vi "General Error Handler CORE.vi"(0 "[error code] (0)":i32 format="%0.0f", 1 "[user-defined codes]":i32[](array[numeric]), 2 "[user-defined descriptions]":string[](array[string]), 5 "[error source] (\" \")":string, 7 "String to Format (not a refnum)":refnum<vi>, 9 "type of dialog (OK msg:1)":T2=enum."OK message", 11 "error in (no error)":errorcluster, 12 "[exception action] (none:0)":i32(ring) items=["no exception", "cancel error on match", "set error on match"], 13 "[exception code]":i32 format="%0.0f", 14 "[exception source]":string) -> (3 "stop event propagated":bool, 4 "error?":bool, 6 "code out":i32 format="%0.0f", 8 "source out":string, 10 "message":string=" INSTRUCTIONS:\r\rNormal Use:  When using subVIs that incorporate the error in/error out (or error I/O) structure, place this handler where you want to inform the user of an error, typically at the end of the I/O data path, as the last action of the program.  If the error in error? is ERROR, the handler creates a message describing the error and its source.  If the type of dialog = 1 (default), the message is displayed to the user, who can only acknowledge it.  If the type = 2, the user can acknowledge the message or abort execution; aborting a program with active I/O is not recommended.  If the type = 0, no message is displayed; this is used to process the error programmatically, and the error out cluster elements are wired to individual terminals for that reason.  \r\rOther Use:\n\r\nlocal testing.  To test the error code of a subVI or function that does not have the error I/O structure, you can wire its error code and a source string to the local error code and error source inputs.  If error in error? indicates no error and error code is not equal to 0, the local code and source are substituted for the error in values, and error? is set TRUE (ERROR).", 15 "error out":errorcluster)   [LabVIEW 2011]
doc: "Indicates whether an error occurred. If an error occurred, this VI returns a description of the error and optionally displays a dialog box."
uses:
  DialogTypeEnum.ctl
  whitespace.ctl
panel:
  in  "prompts":T1={"Error %d occurred at %s"="Error %d occurred at %s", "Warning %d occurred at %s"="Warning %d occurred at %s", "Possible reasons: %s"="<b>Possible reason(s):</b>\\n%s", "Error not listed"="This error code is undefined. Undefined errors might occur for a number of reasons. For example, no one has provided a description for the code, or you might have wired a number that is not an error code to the error code input. \n\nAdditionally, undefined error codes might occur because the error relates to a third-party object, such as the operating system or ActiveX. For these third-party errors, you might be able to obtain a description of the error by searching the Web for the error code (%s) or for its hexadecimal representation (0x%s).", "GetCommError x%lx"="Windows GetCommError:  The hex value of this code is <B>x%04lx</B>.\n\nInterpret it bit-wise as follows:\n<B>x4000</B>: serial port VI error\n<B>x0001</B>: receiving queue overflowed or character was received after end-of-file character\n<B>x0002</B>: character was lost by overwrite\n<B>x0004</B>: parity error\n<B>x0008</B>: framing error\n<B>x0010</B>: break condition\n<B>x0020</B>: CTS timeout\n<B>x0040</B>: DSR timeout\n<B>x0080</B>: RLSD timeout\n<B>x0100</B>: transmission queue was full when new character arrived\n<B>x0200</B>: parallel device timeout\n<B>x0400</B>: parallel device I/O error\n<B>x0800</B>: parallel device not selected\n<B>x1000</B>: parallel device out of paper\n<B>x8000</B>: requested mode is  not supported or the idComDev parameter is invalid.", "Continue"="Continue", "Stop"="Stop", "an unidentified location"="an unidentified location", "No Error"="No Error", "Help"="Why not found?"}
  # "reinitialize to default to display instructions"
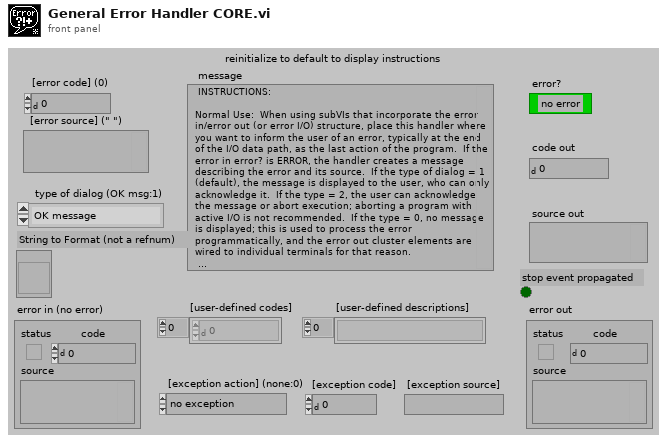
[diagram p1: front panel]
types:
  T1 = cluster{"Error %d occurred at %s":string, "Warning %d occurred at %s":string, "Possible reasons: %s":string, "Error not listed":string, "GetCommError x%lx":string, "Continue":string, "Stop":string, "an unidentified location":string, "No Error":string, "Help":string}
  T2 = typedef "DialogTypeEnum.ctl" = enum16{"no dialog", "OK message", "continue or stop message", "auto error handling dialog", "OK message + warnings", "continue/stop + warnings"}
  T3 = typedef "TagReturnType.ctl" = enum16{"No Tag", "<err>", "<append>"}
  T4 = typedef "whitespace.ctl" = u16
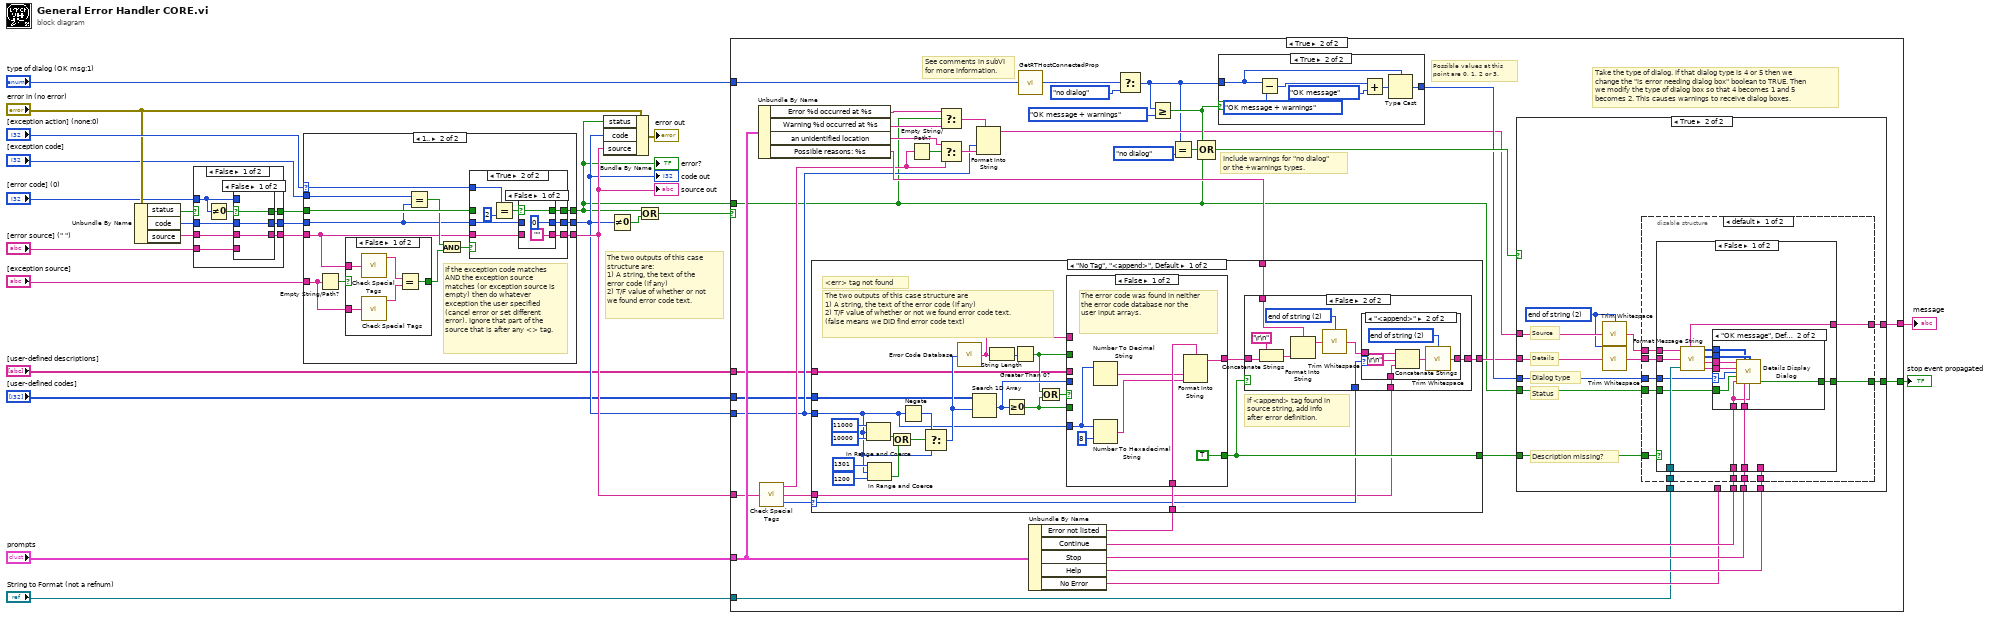
[diagram p0: block diagram]
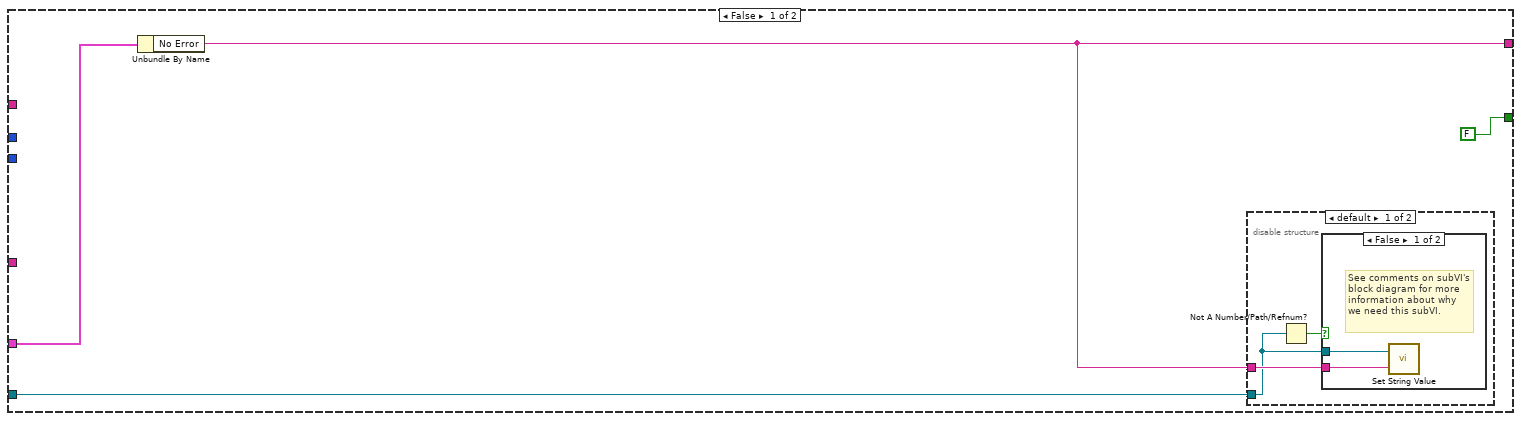
[diagram p8: hidden frame]
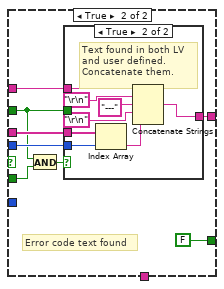
[diagram p14: hidden frame]
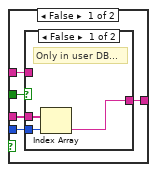
[diagram p15: hidden frame]
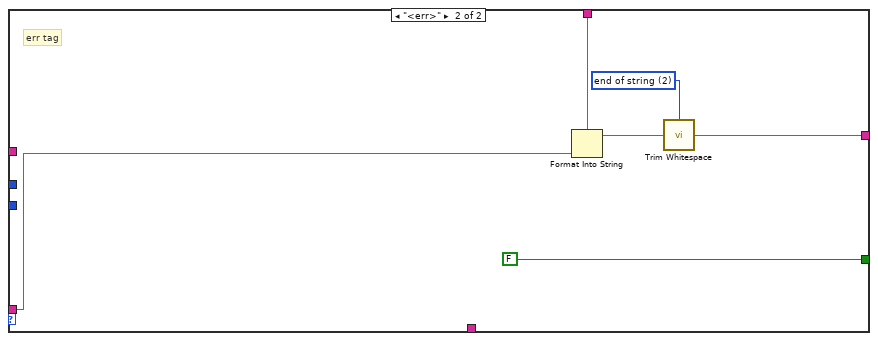
[diagram p17: hidden frame]
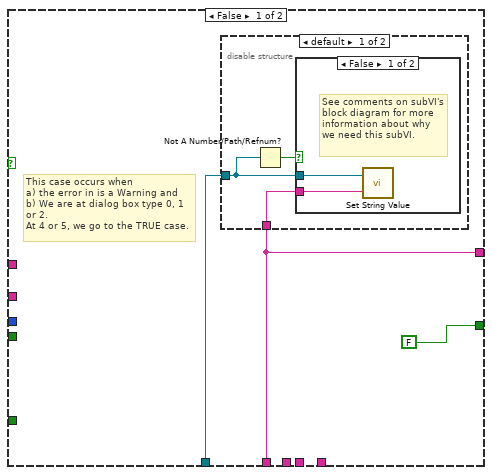
[diagram p18: hidden frame]
diagram:
  # "The two outputs of this case structure are:\n1) A string, the text of the error code (if any)\n2) T/F value of whether or not we found error code text."
  n1 = Unbundle By Name("error in (no error)") -> ("status"=w6:bool, "code"=w20:i32, "source"=w24:string)
  n2 = case shown="False" w6 {
    selector: w6 -> [_ w42]
    tunnel: [w31 w41] -> w22
    tunnel: [w32 w42] -> w21
    tunnel: w20 -> [w28 w41]
    tunnel: [w30 w40] -> w23
    tunnel: w24 -> [w29 w40]
    tunnel: "[error code] (0)" -> [w27 _]
    tunnel: "[error source] (\" \")" -> [w26 _]
    frame False {
      n3 = Not Equal To 0?(x=w27) -> (x != 0?=w33:bool)
      n4 = case shown="False" w33 {
        selector: w33 -> [w36 w39]
        tunnel: [w36 w39] -> w32
        tunnel: w27 -> [_ w38]
        tunnel: [w34 w38] -> w31
        tunnel: w26 -> [_ w37]
        tunnel: [w35 w37] -> w30
        tunnel: w29 -> [w35 _]
        tunnel: w28 -> [w34 _]
        frame False {
        }
        frame True {
        }
      }
    }
    frame True {
    }
  }
  n5 = case shown="1.." "[exception action] (none:0)" {
    selector: "[exception action] (none:0)" -> [_ w50]
    tunnel: [w45 w58] -> w2
    tunnel: w21 -> [w45 w56]
    tunnel: [w44 w57] -> w7
    tunnel: w22 -> [w44 w54]
    tunnel: [w43 w52] -> w17
    tunnel: w23 -> [w43 w48]
    tunnel: "[exception code]" -> [_ w51]
    tunnel: "[exception source]" -> [_ w47]
    frame ..0 {
    }
    frame 1.. {
      # "If the exception code matches AND the exception source matches (or exception source is empty) then do whatever exception the user specified (cancel error or set different error). Ignore that part of the source that is after any <> tag."
      n6 = Empty String/Path?(string/path=w47) -> (empty?=w49:bool)
      n7 = case shown="False" w49 {
        selector: w49 -> [_ w64]
        tunnel: w48 -> [w63 _]
        tunnel: w47 -> [w62 _]
        tunnel: [w61 w64] -> w46
        frame False {
          n8 = call "Check Special Tags.vi"("source"=w63) -> ("Before Tag (source)"=w60:string)  [unwired: 2 out]
          n9 = call "Check Special Tags.vi"("source"=w62) -> ("Before Tag (source)"=w59:string)  [unwired: 2 out]
          n10 = Equal?(x=w60, y=w59) -> (x = y?=w61:bool)
        }
        frame True {
          # "Empty string always matches."
        }
      }
      n11 = Equal?(x=w51, y=w54) -> (x = y?=w55:bool)
      n12 = And(x=w55, y=w46) -> (x .and. y?=w53:bool)
      n13 = case shown="True" w53 {
        tunnel: [w67 w68] -> w58
        tunnel: [w66 w72] -> w57
        tunnel: w56 -> [w67 _]
        tunnel: w54 -> [w66 w71]
        tunnel: w50 -> [_ w75]
        tunnel: [w65 w70] -> w52
        tunnel: w48 -> [w65 w69]
        frame False {
        }
        frame True {
          n14 = Equal?(x=w75, y=2) -> (x = y?=w73:bool)
          n15 = case shown="False" w73 {
            selector: w73 -> [w78 w81]
            tunnel: [0 w80] -> w72
            tunnel: w71 -> [_ w80]
            tunnel: ["" ("Empty String Constant") w79] -> w70
            tunnel: w69 -> [_ w79]
            tunnel: [w78 w81] -> w68
            frame False {
            }
            frame True {
            }
          }
        }
      }
    }
  }
  "source out" <- w17
  "error?" <- w2
  "code out" <- w7
  n16 = Bundle By Name(cluster="error in (no error)", "status"=w2, "code"=w7, "source"=w17) -> (→"error out":errorcluster)
  n17 = Not Equal To 0?(x=w7) -> (x != 0?=w1:bool)
  n18 = Or(x=w2, y=w1) -> (x .or. y?=w18:bool)
  n19 = case shown="True" w18 {
    tunnel: [w83 w109] -> w25
    tunnel: w2 -> [_ w91]
    tunnel: w17 -> [_ w99]
    tunnel: "prompts" -> [w85 w118]
    tunnel: [FALSE ("Stop 2") w112] -> w13
    tunnel: "String to Format (not a refnum)" -> [w82 w105]
    tunnel: w7 -> [_ w97]
    tunnel: "[user-defined descriptions]" -> [_ w95]
    tunnel: "[user-defined codes]" -> [_ w94]
    tunnel: "type of dialog (OK msg:1)" -> [_ w93]
    frame False {
      n20 = Unbundle By Name(w85) -> ("No Error"=w83:string)
      n21 = disable-structure shown="default" {
        disable-tunnel: w83 -> [w88 _]
        disable-tunnel: w82 -> [w87 _]
        frame condition #0 (active) {
          n22 = Not A Number/Path/Refnum?(number/path/refnum=w87) -> (NaN/Path/Refnum?=w86:bool)
          n23 = case shown="False" w86 {
            tunnel: w88 -> [w90 _]
            tunnel: w87 -> [w89 _]
            frame False {
              # "See comments on subVI's block diagram for more information about why we need this subVI."
              n24 = call "Set String Value.vi"("No Error"=w90, "String to Format (not a refnum)"=w89) -> ()
            }
            frame True {
            }
          }
        }
        frame condition #1 {
          # "Do nothing in RT case."
        }
      }
    }
    frame True {
      # "See comments in subVI for more information."
      # "Include warnings for \"no dialog\" or the +warnings types."
      # "Possible values at this point are 0, 1, 2 or 3."
      # "Take the type of dialog. If that dialog type is 4 or 5 then we change the \"is error needing dialog box\" boolean to TRUE. Then we modify the type of dialog box so that 4 becomes 1 and 5 becomes 2. This causes warnings to receive dialog boxes."
      n25 = Unbundle By Name(w118) -> ("Error %d occurred at %s"=w96:string, "Warning %d occurred at %s"=w125:string, "an unidentified location"=w122:string, "Possible reasons: %s"=w111:string)
      n26 = call "Check Special Tags.vi"("source"=w99) -> ("Before Tag (source)"=w98:string, "After Tag (special data)"=w126:string, "Tag Found?"=w113:T3)
      n27 = Empty String/Path?(string/path=w98) -> (empty?=w127:bool)
      n28 = Select(t=w96, s=w91, f=w125) -> (s? t:f=w124:string)
      n29 = Select(t=w122, s=w127, f=w98) -> (s? t:f=w123:string)
      n30 = Format Into String(format string=w124, w97, w123) -> (resulting string=w107:string)  [unwired: 2 in, 1 out]
      n31 = call "GetRTHostConnectedProp.vi"() -> ("App.RTHostConnected"=w92:bool)
      n32 = Unbundle By Name(w118) -> ("Error not listed"=w121:string, "Continue"=w120:string, "Stop"=w119:string, "Help"=w116:string, "No Error"=w106:string)
      n33 = case shown="\"No Tag\", \"<append>\", Default" w113 {
        selector: w113 -> [w141 _]
        tunnel: [w139 w213] -> w108
        tunnel: w97 -> [w135 _]
        tunnel: w126 -> [w140 w212]
        tunnel: w121 -> [w159 _]
        tunnel: [w142 FALSE] -> w117
        tunnel: w111 -> [w144 w211]
        tunnel: w95 -> [w137 _]
        tunnel: w94 -> [w136 _]
        frame "No Tag", "<append>", Default {
          # "If <append> tag found in source string, add info after error definition."
          # "<err> tag not found"
          # "The two outputs of this case structure are\n1) A string, the text of the error code (if any)\n2) T/F value of whether or not we found error code text.\n(false means we DID find error code text)"
          n34 = In Range and Coerce(upper limit=11000, x=w135, lower limit=10000) -> (In Range?=w152:bool)  [unwired: 1 out]
          n35 = In Range and Coerce(upper limit=1301, x=w135, lower limit=1200) -> (In Range?=w153:bool)  [unwired: 1 out]
          n36 = Or(x=w152, y=w153) -> (x .or. y?=w151:bool)
          n37 = Negate(x=w135) -> (-x=w155:i32)
          n38 = Select(t=w155, s=w151, f=w135) -> (s? t:f=w138:i32)
          n39 = call "Error Code Database.vi"("Error Code"=w138) -> ("Error Text"=w145:string)
          n40 = Search 1D Array(1D array=w136, element=w138) -> (index of element=w158:i32)  [unwired: 1 in]
          n41 = String Length(string=w145) -> (length=w149:i32)
          n42 = Greater Or Equal To 0?(x=w158) -> (x >= 0?=w146:bool)
          n43 = Greater Than 0?(x=w149) -> (x > 0?=w147:bool)
          n44 = Or(x=w147, y=w146) -> (x .or. y?=w148:bool)
          n45 = case shown="False" w148 {
            tunnel: w158 -> [_ w188]
            tunnel: [w182 w186] -> w143
            tunnel: w159 -> [w181 _]
            tunnel: [TRUE FALSE] -> w142
            tunnel: w147 -> [_ w185]
            tunnel: w146 -> [_ w190]
            tunnel: w137 -> [_ w189]
            tunnel: w145 -> [_ w187]
            tunnel: w135 -> [w178 _]
            frame False {
              # "The error code was found in neither the error code database nor the user input arrays."
              n46 = Number To Decimal String(number=w178) -> (decimal integer string=w179:string)  [unwired: 1 in]
              n47 = Number To Hexadecimal String(1:i16 8 ("width (-)"), 2:w178) -> (0:w180:string)
              n48 = Format Into String(format string=w181, w179, w180) -> (resulting string=w182:string)  [unwired: 2 in, 1 out]
            }
            frame True {
              # "Error code text found"
              n49 = And(x=w185, y=w190) -> (x .and. y?=w191:bool)
              n50 = case shown="True" w191 {
                tunnel: w189 -> [w194 w209]
                tunnel: w188 -> [w193 w208]
                tunnel: w187 -> [w195 w202]
                tunnel: [w196 w206] -> w186
                tunnel: w185 -> [w197 _]
                frame False {
                  n51 = case shown="False" w197 {
                    tunnel: [w198 w201] -> w196
                    tunnel: w195 -> [_ w201]
                    tunnel: w194 -> [w200 _]
                    tunnel: w193 -> [w199 _]
                    frame False {
                      # "Only in user DB..."
                      n52 = Index Array(array=w200, index=w199) -> (element=w198:string)
                    }
                    frame True {
                      # "Only in LV DB..."
                    }
                  }
                }
                frame True {
                  # "Text found in both LV\nand user defined. \nConcatenate them."
                  n53 = Index Array(array=w209, index=w208) -> (element=w207:string)
                  n54 = Concatenate Strings(w202, "\r\n" ("End of Line Constant"), "---" ("string"), "\r\n" ("End of Line Constant"), w207) -> (w206:string)
                }
              }
            }
          }
          n55 = case shown="False" w142 {
            tunnel: w144 -> [_ w170]
            tunnel: [w160 w162] -> w139
            tunnel: w143 -> [w160 w167]
            tunnel: w141 -> [_ w164]
            tunnel: w140 -> [_ w163]
            frame True {
              # "no explanation given for error."
            }
            frame False {
              w161 = T4 2 items=["both", "start of string", "end of string"] ("location (both)")
              n56 = Concatenate Strings("\r\n" ("End of Line Constant"), w167) -> (w168:string)
              n57 = Format Into String(format string=w170, w168) -> (resulting string=w169:string)  [unwired: 2 in, 1 out]
              n58 = call "Trim Whitespace.vi"("string"=w169, "location (both)"=w161) -> ("trimmed string"=w165:string)
              n59 = case shown="\"<append>\"" w164 {
                tunnel: w165 -> [w171 w176]
                tunnel: [w171 w173] -> w162
                tunnel: w163 -> [_ w175]
                frame "No Tag", Default {
                }
                frame "<append>" {
                  w172 = T4 2 items=["both", "start of string", "end of string"] ("location (both)")
                  n60 = Concatenate Strings(w176, "\r\n" ("End of Line Constant"), w175) -> (w174:string)
                  n61 = call "Trim Whitespace.vi"("string"=w174, "location (both)"=w172) -> ("trimmed string"=w173:string)
                }
              }
            }
          }
        }
        frame "<err>" {
          w210 = T4 2 items=["both", "start of string", "end of string"] ("location (both)")
          # "err tag"
          n62 = Format Into String(format string=w211, w212) -> (resulting string=w214:string)  [unwired: 2 in, 1 out]
          n63 = call "Trim Whitespace.vi"("string"=w214, "location (both)"=w210) -> ("trimmed string"=w213:string)
        }
      }
      n64 = Select(t=w93, s=w92, f=DialogTypeEnum."no dialog" ("type of dialog (OK msg:1)")) -> (s? t:f=w100:T2)
      n65 = Greater Or Equal?(x=w100, y=DialogTypeEnum."OK message + warnings" ("type of dialog (OK msg:1)")) -> (x >= y?=w114:bool)
      n66 = Equal?(x=w100, y=DialogTypeEnum."no dialog" ("type of dialog (OK msg:1)")) -> (x = y?=w104:bool)
      n67 = Compound Arithmetic op=OR(w114, w104, w91) -> (w115:bool)
      n68 = case shown="True" w114 {
        tunnel: w100 -> [w128 w129]
        tunnel: [w128 w131] -> w110
        frame False {
        }
        frame True {
          n69 = Subtract(x=w129, y=DialogTypeEnum."OK message + warnings" ("type of dialog (OK msg:1)")) -> (x-y=w134:u16)
          n70 = Add(x=w134, y=DialogTypeEnum."OK message" ("type of dialog (OK msg:1)")) -> (x+y=w130:u16)
          n71 = Type Cast(type=w129, x=w130) -> (*(type *) &x=w131:T2)
        }
      }
      n72 = case shown="True" w115 {
        tunnel: w110 -> [_ w237]
        tunnel: w120 -> [_ w236]
        tunnel: w119 -> [_ w235]
        tunnel: w117 -> [_ w224]
        tunnel: w116 -> [_ w234]
        tunnel: w107 -> [_ w227]
        tunnel: w108 -> [_ w228]
        tunnel: w91 -> [_ w233]
        tunnel: [FALSE ("Stop 2") w232] -> w112
        tunnel: [w216 w231] -> w109
        tunnel: w106 -> [w216 _]
        tunnel: w105 -> [w217 w230]
        frame False {
          # "This case occurs when\na) the error in is a Warning and\nb) We are at dialog box type 0, 1 or 2.\nAt 4 or 5, we go to the TRUE case."
          n73 = disable-structure shown="default" {
            disable-tunnel: w217 -> [w221 _]
            disable-tunnel: w216 -> [w219 _]
            frame condition #0 (active) {
              n74 = Not A Number/Path/Refnum?(number/path/refnum=w221) -> (NaN/Path/Refnum?=w220:bool)
              n75 = case shown="False" w220 {
                tunnel: w219 -> [w223 _]
                tunnel: w221 -> [w222 _]
                frame False {
                  # "See comments on subVI's block diagram for more information about why we need this subVI."
                  n76 = call "Set String Value.vi"("No Error"=w223, "String to Format (not a refnum)"=w222) -> ()
                }
                frame True {
                }
              }
            }
            frame condition #1 {
              # "Do nothing in RT case."
            }
          }
        }
        frame True {
          w225 = T4 2 items=["both", "start of string", "end of string"] ("location (both)")
          # "Description missing?"
          # "Dialog type"
          # "Status"
          # "Details"
          # "Source"
          n77 = call "Trim Whitespace.vi"("string"=w227, "location (both)"=w225) -> ("trimmed string"=w226:string)
          n78 = call "Trim Whitespace.vi"("string"=w228, "location (both)"=w225) -> ("trimmed string"=w229:string)
          n79 = disable-structure "Conditional Disable Structure" shown="default" {
            disable-tunnel: w237 -> [w248 w292]
            disable-tunnel: w236 -> [w247 w291]
            disable-tunnel: w235 -> [w246 w290]
            disable-tunnel: w234 -> [w245 _]
            disable-tunnel: w233 -> [w244 _]
            disable-tunnel: [w243 w289] -> w232
            disable-tunnel: [w242 w288] -> w231
            disable-tunnel: w230 -> [w241 w287]
            disable-tunnel: w229 -> [w240 w286]
            disable-tunnel: w226 -> [w239 w285]
            disable-tunnel: w224 -> [w238 _]
            frame condition #0 (active) {
              n80 = case shown="False" w238 {
                tunnel: w240 -> [w260 w276]
                tunnel: w245 -> [_ w282]
                tunnel: w247 -> [w256 w280]
                tunnel: w246 -> [w255 w279]
                tunnel: w248 -> [w258 w281]
                tunnel: [w257 w278] -> w243
                tunnel: w239 -> [w261 w277]
                tunnel: w244 -> [w254 _]
                tunnel: [w249 w274] -> w242
                tunnel: w241 -> [w259 w272]
                frame False {
                  n81 = call "Format Message String.vi"("Source"=w261, "Details"=w260, "String to Format (not a refnum)"=w259) -> ("message"=w249:string, "Bold Start"=w253:i32[], "Bold Length"=w252:i32[], "Source Out"=w251:string, "Details Out"=w250:string)  [unwired: 1 in]
                  n82 = case shown="\"OK message\", Default" w258 {
                    selector: w258 -> [_ w268]
                    tunnel: [FALSE ("stop event propagated") w271] -> w257
                    tunnel: w256 -> [_ w269]
                    tunnel: w255 -> [_ w270]
                    tunnel: w254 -> [_ w267]
                    tunnel: w253 -> [_ w263]
                    tunnel: w252 -> [_ w266]
                    tunnel: w251 -> [_ w265]
                    tunnel: w250 -> [_ w264]
                    frame "no dialog" {
                    }
                    frame "OK message", Default {
                      n83 = call "Details Display Dialog.vi"("Source"=w265, "Start"=w263, "Length"=w266, "Details"=w264, "dialog type"=w268, "Error or Warning"=w267, "contname"=w269, "stopname"=w270, "okname"=w269) -> ("stop event propagated"=w271:bool)  [unwired: 6 in]
                    }
                  }
                }
                frame True {
                  w275 = "\r\n" ("End of Line Constant")
                  n84 = Concatenate Strings(w277, w275, w275, w276) -> (w274:string)
                  n85 = Not A Number/Path/Refnum?(number/path/refnum=w272) -> (NaN/Path/Refnum?=w273:bool)
                  n86 = call "Not Found Dialog.vi"("Help"=w282, "Message"=w274, "Stop"=w279, "Continue"=w280, "type of dialog (OK msg:1)"=w281) -> ("stop event propagated"=w278:bool)  [unwired: 1 in]
                  n87 = case shown="False" w273 {
                    tunnel: w272 -> [w284 _]
                    tunnel: w274 -> [w283 _]
                    frame False {
                      n88 = call "Set String Value.vi"("No Error"=w283, "String to Format (not a refnum)"=w284) -> ()
                    }
                    frame True {
                    }
                  }
                }
              }
            }
            frame condition #1 {
              n89 = call "Format Message String.vi"("Source"=w285, "Details"=w286, "String to Format (not a refnum)"=w287) -> ("message"=w288:string)  [unwired: 1 in, 4 out]
              n90 = case shown="\"continue or stop message\", \"continue/stop + warnings\"" w292 {
                tunnel: [FALSE ("stop event propagated") FALSE ("stop event propagated") FALSE ("stop event propagated") w303] -> w289
                tunnel: w288 -> [_ w295 w302 w307]
                tunnel: w291 -> [_ w294 w301 w306]
                tunnel: w290 -> [_ _ w300 w305]
                frame "no dialog" {
                }
                frame "OK message", "OK message + warnings", Default {
                  n91 = One Button Dialog(message=w295, button name ("OK")=w294) -> ()  [unwired: 1 out]
                }
                frame "continue or stop message", "continue/stop + warnings" {
                  n92 = Two Button Dialog(message=w302, 1:w300, 2:w301) -> (T button?=w298:bool)
                  n93 = Not(x=w298) -> (.not. x?=w297:bool)
                  n94 = Stop(stop? (T)=w297) -> ()
                }
                frame "auto error handling dialog" {
                  n95 = Two Button Dialog(message=w307, 1:w305, 2:w306) -> (T button?=w304:bool)
                  n96 = Not(x=w304) -> (.not. x?=w303:bool)
                }
              }
            }
          }
        }
      }
    }
  }
  "message" <- w25
  "stop event propagated" <- w13
